vi "DSF.Engine.Transfer Static Method 11.vi"(8 "error in (no error)":errorcluster, 11 "Transfer in":refnum<class "DSF.Engine.Transfer.lvclass">) -> (0 "error out":errorcluster, 3 "Transfer out":refnum<class "DSF.Engine.Transfer.lvclass">)   [LabVIEW 2017, in "DSF.Engine.lvlib" / "DSF.Engine.Transfer.lvclass"]
uses:
  DSF.Engine.Transfer.lvclass
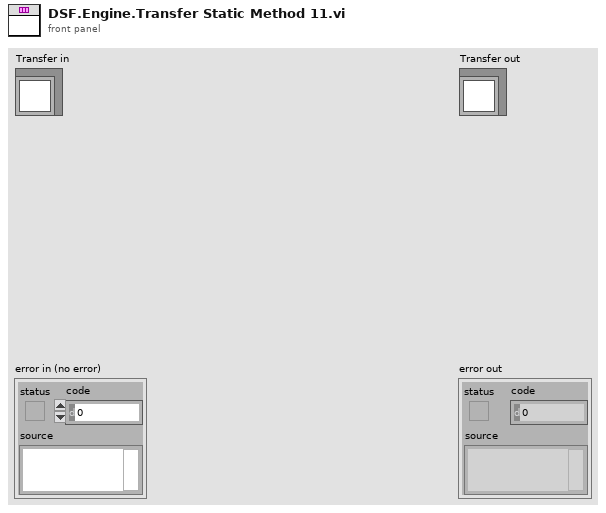
[diagram p1: front panel]
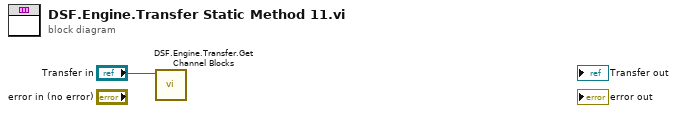
[diagram p0: block diagram]
diagram:
  n1 = call "DSF.Engine.Transfer.Get Channel Blocks.vi"("Transfer in"="Transfer in") -> ()  [unwired: 9 in, 2 out]
